vi "Exemple 3.vi"() -> ()   [LabVIEW 2021]
uses:
  C:/Users/Phalanx/Documents/LUGE/ExempleLUGE/bin/Release/ExempleLUGE.dll
  Documents/LUGE/ExempleLUGE/bin/Release/ExempleLUGE.dll
panel:
  in  "Threshold":i32=20
  out "error out":errorcluster
  in  "Max":i32=50
  in  "ProgressBarWithLabel":refnum<k24>(container)
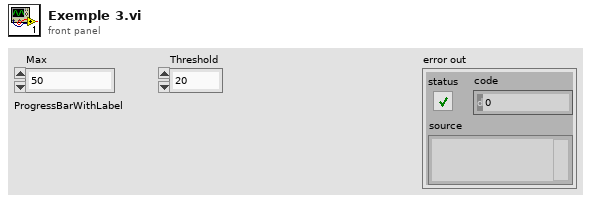
[diagram p1: front panel]
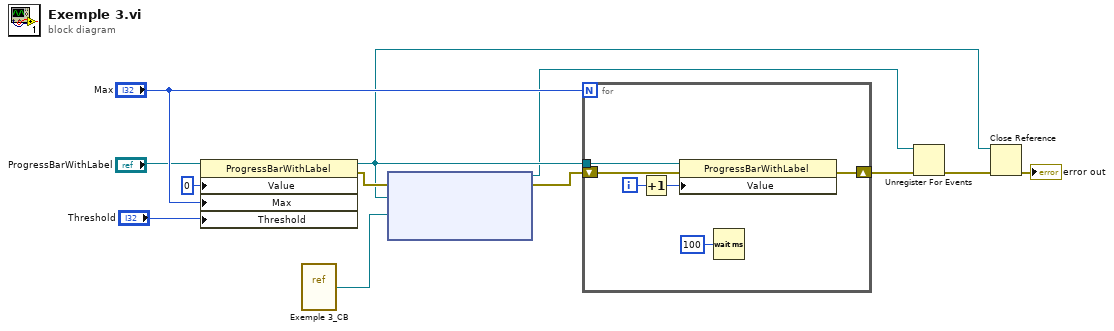
[diagram p0: block diagram]
diagram:
  n1 = property class="ProgressBarWithLabel"(reference="ProgressBarWithLabel", "Value"=0, "Max"="Max", "Threshold"="Threshold") -> (reference out=w5:refnum<k24>, error out=w7:errorcluster)  [unwired: 1 in]
  n2 = vi-ref "Exemple 3_CB.vi"() -> ("vi reference"=w4:refnum<vi>)
  n3 = node(w7, w5, w4) -> (w1:refnum<k27>, w6:errorcluster)  [unwired: 2 in]
  n4 = for {
    N: "Max" -> [_]
    tunnel: w5 -> [w18]
    shift-right: [w14] -> w3
    shift-left: w6 -> [w15]
    i -> [w17]
    n5 = Increment(x=w17) -> (x+1=w16:i32)
    n6 = property class="ProgressBarWithLabel"(reference=w18, error in=w15, "Value"=w16) -> (error out=w14:errorcluster)  [unwired: 1 out]
    n7 = Wait (ms)(milliseconds to wait=u32 100) -> ()  [unwired: 1 out]
  }
  n8 = Unregister For Events(event registration refnum=w1, error in=w3) -> (error out=w2:errorcluster)
  n9 = Close Reference(reference=w5, error in (no error)=w2) -> (error out=→"error out":errorcluster)
